vi "OMR.vi"(0 "System no.":i32=1 min=1 max=4 step=1, 2 "Axes to move":string[](array[string]), 3 "Position values":dbl[](array[numeric]) format="%.6f", 4 "No.of digits":i16=4, 5 "error in":errorcluster) -> (19 "error out":errorcluster)   [LabVIEW 2020]
doc: "Open-loop move relative. Sets new relative open-loop target position for given axes. Servo must be disabled for all commanded axes prior to using this command.\n\nE-861: This command works only in open-loop operation. With closed-loop systems, use MVR instead to command motion. Do not call OMA or OMR for axes which have no sensor, otherwise stage will run into hard stop. Motion commands are not allowed when a joystick is active on the axis. OMR can not be processed as long as motion commanded by a former OMR or OMA command is still performed.\n\nE-871, E-873: This command works only in open-loop operation. With closed-loop systems, use MOV instead to command motion. Do not call OMA or OMR for axes which have no sensor, otherwise stage will run into hard stop. Motion commands are not allowed when a joystick is active on the axis."
panel:
  # "Open-loop Move Relative. Sets new relative open-loop target \nposition for given axes."
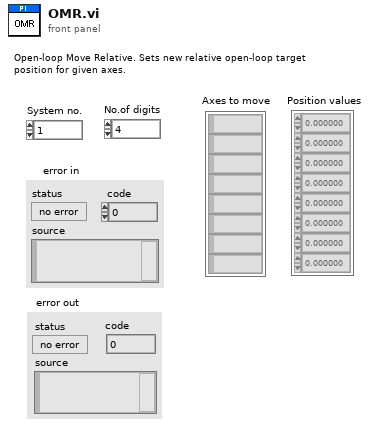
[diagram p1: front panel]
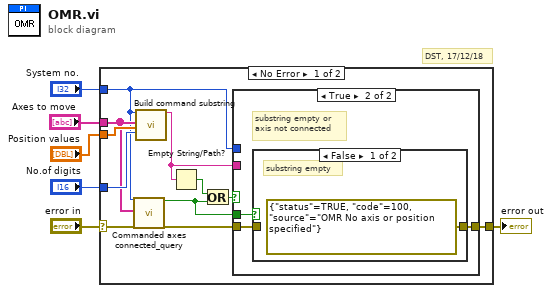
[diagram p0: block diagram]
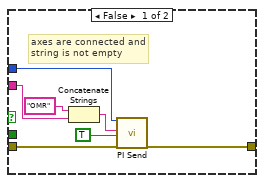
[diagram p2: hidden frame]
diagram:
  # "DST, 17/12/18"
  n1 = case shown="No Error" "error in" {
    selector: "error in" -> [w8 w30]
    tunnel: [w17 w30] -> w6
    tunnel: "Position values" -> [w16 _]
    tunnel: "No.of digits" -> [w15 _]
    tunnel: "System no." -> [w7 _]
    tunnel: "Axes to move" -> [w13 _]
    frame No Error {
      n2 = call "Commanded axes connected_query.vi"("System no."=w7, "Commanded axes"=w13, "error in"=w8) -> ("Controller error"=w11:bool, "error out"=w14:errorcluster)  [unwired: 1 in, 14 out]
      n3 = call "Build command substring.vi"("System no."=w7, "Affected axes"=w13, "Parameters"=w16, "No. of digits"=w15) -> ("Command substring"=w9:string)  [unwired: 3 in, 12 out]
      n4 = Empty String/Path?(string/path=w9) -> (empty?=w10:bool)
      n5 = Or(x=w10, y=w11) -> (x .or. y?=w12:bool)
      n6 = case shown="True" w12 {
        tunnel: w9 -> [w23 _]
        tunnel: [w19 w27] -> w17
        tunnel: w14 -> [w20 w25]
        tunnel: w11 -> [_ w26]
        tunnel: w7 -> [w18 _]
        frame False {
          # "axes are connected and\nstring is not empty"
          n7 = Concatenate Strings("OMR", w23) -> (w21:string)
          n8 = call "PI Send.vi"("System no."=w18, "String to send"=w21, "Attach termination char.?"=TRUE ("Attach Linefeed?"), "error in"=w20) -> ("error out"=w19:errorcluster)  [unwired: 2 in, 13 out]
        }
        frame True {
          # "substring empty or\naxis not connected"
          n9 = case shown="False" w26 {
            tunnel: [errorcluster {"status"=TRUE, "code"=100, "source"="OMR No axis or position specified"} ("error out") w29] -> w27
            tunnel: w25 -> [_ w29]
            frame False {
              # "substring empty"
            }
            frame True {
              # "commanded axis\nnot connected"
            }
          }
        }
      }
    }
    frame Error {
    }
  }
  "error out" <- w6
